vi "initialise.vi"(8 "error in (no error)":errorcluster, 11 "FPGA_AK101022Resonance in":refnum<class "FPGAWrapperAK101022Resonance.lvclass">) -> (0 "error out":errorcluster, 3 "FPGA_AK101022Resonance out":refnum<class "FPGAWrapperAK101022Resonance.lvclass">)   [LabVIEW 2010, in "FPGAWrapperAK101022Resonance.lvclass"]
uses:
  FPGAWrapperAK101022Resonance.lvclass
  GenericFPGAWrapper/GenericFPGAWrapper/GenericFPGAWrapper.lvclass
  scan_specification_cluster.ctl
  grabber/config_data_cluster.ctl
  FPGAWrapperAK101022Resonance.lvclass/FPGAWrapperAK101022Resonance.ctl
  class_data.vi
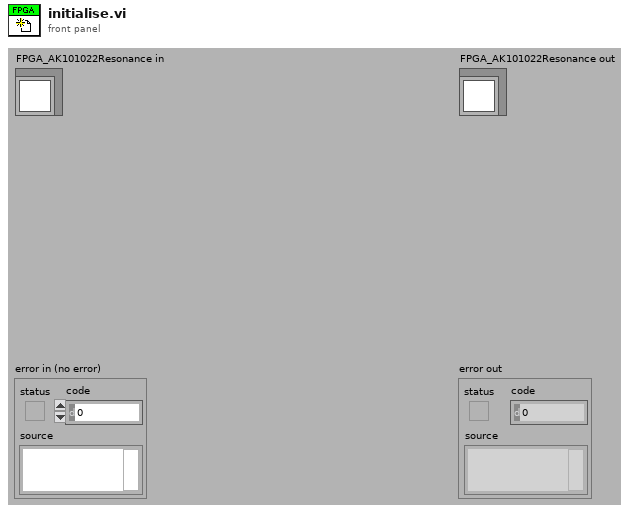
[diagram p1: front panel]
types:
  T1 = typedef "scan_specification_cluster.ctl" = cluster{"x amplitude":u16, "x resolution (pixels)":u16, "x offset fly-forward (iterations)":u16, "x offset fly-back (iterations)":u16, "y resolution (nr. of lines)":u16, "y step size":u16, "iterations per pixel":u16, "number of frames":i32, "y offset (pixels)":u16, "number of y-brake lines  (before y-fly-back)":u16, "number y-brake lines (after y-fly-back)":u16, "number of y-fly-back steps":u16, "lines per z step":u16, "number of z/intensity tuples":u16}
  T2 = typedef "config_data_cluster.ctl" = cluster{"channel offsets":u32[], "invert channel?":bool[], "ADC clock phase":i32}
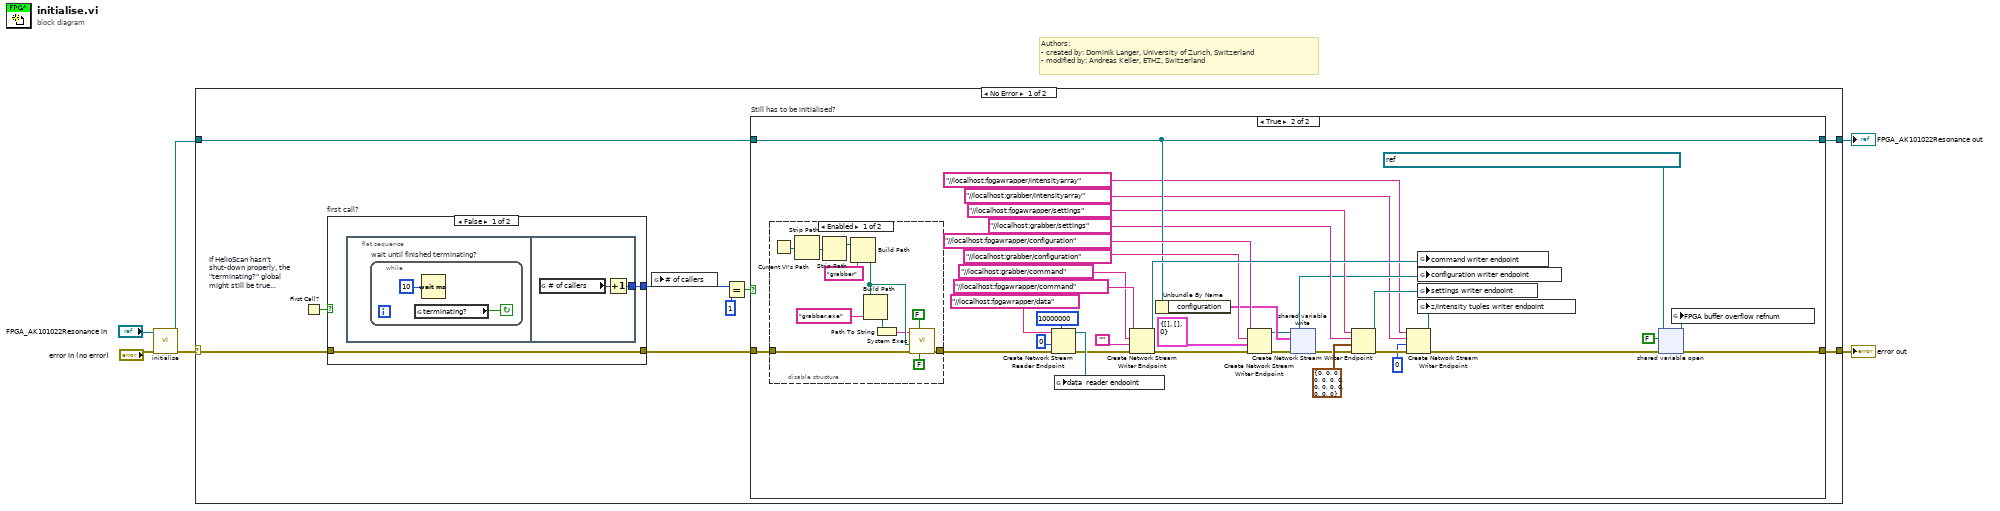
[diagram p0: block diagram]
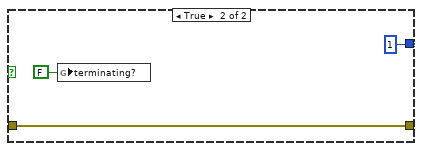
[diagram p2: hidden frame]
diagram:
  # "Authors: \n- created by: Dominik Langer, University of Zurich, Switzerland\n- modified by: Andreas Keller, ETHZ, Switzerland"
  n1 = call-parent "initialise.vi"("error in (no error)"="error in (no error)", "GenericPlugin in"="FPGA_AK101022Resonance in") -> ("error out"=w2:errorcluster, "GenericPlugin out"=w1:refnum<class "FPGAWrapperAK101022Resonance.lvclass">)  [unwired: 8 in]
  n2 = case shown="No Error" w2 {
    selector: w2 -> [w8 w76]
    tunnel: [w15 w76] -> w6
    tunnel: w1 -> [w7 w75]
    tunnel: [w9 w75] -> w5
    frame No Error {
      n3 = First Call? "If HelioScan hasn't shut-down properly, the \"terminating?\" global might still be true..."() -> (First Call?: T/F=w14:bool)
      n4 = case "first call?" shown="False" w14 {
        tunnel: [w17 1 ("# of callers")] -> w12
        tunnel: [w16 w23] -> w13
        tunnel: w8 -> [w16 w23]
        frame False {
          n5 = flat-sequence {
            tunnel: [w21] -> w17
            frame #0 {
              n6 = while "wait until finished terminating?" {
                stop <- w18 continue-if-true
                n7 = global read "class_data.vi" "terminating?"() -> (w18:bool)
                n8 = Wait (ms)(milliseconds to wait=u32 10) -> ()  [unwired: 1 out]
              }
            }
            frame #1 {
              n9 = global read "class_data.vi" "# of callers"() -> (w20:i32)
              n10 = Increment(x=w20) -> (x+1=w21:i32)
            }
          }
        }
        frame True {
          n11 = global write "class_data.vi" "terminating?"(FALSE ("terminating?")) -> ()
        }
      }
      n12 = global write "class_data.vi" "# of callers"(w12) -> ()
      n13 = Equal?(x=w12, y=1) -> (x = y?=w10:bool)
      n14 = case "Still has to be initialised?" shown="True" w10 {
        tunnel: w13 -> [w26 w61]
        tunnel: [w26 w45] -> w15
        tunnel: w7 -> [w25 w42]
        tunnel: [w25 w42] -> w9
        frame False {
        }
        frame True {
          n15 = disable-structure shown="Enabled" {
            disable-tunnel: w61 -> [w66 w74]
            disable-tunnel: [w65 w74] -> w53
            frame Enabled {
              n16 = Current VI's Path() -> (path=w64:path)
              n17 = Strip Path(path=w64) -> (stripped path=w63:path)  [unwired: 1 out]
              n18 = Strip Path(path=w63) -> (stripped path=w62:path)  [unwired: 1 out]
              n19 = Build Path(base path=w62, name or relative path="grabber") -> (appended path=w71:path)
              n20 = Build Path(base path=w71, name or relative path="grabber.exe" ("command line")) -> (appended path=w70:path)
              n21 = Path To String(path=w70) -> (string=w69:string)
              n22 = call <vilib>:"System Exec.vi"("run minimized? (F)"=FALSE, "wait until completion? (T)"=FALSE, "error in (no error)"=w66, "working directory"=w71, "command line"=w69) -> ("error out"=w65:errorcluster)  [unwired: 3 in, 3 out]
            }
            frame Disabled {
            }
          }
          n23 = Create Network Stream Reader Endpoint(7:10000000 ("reader buffer size"), 8:w53, 9:u32 0, 11:"//localhost:fpgawrapper/data" ("writer name")) -> (0:w50:errorcluster, 3:w58:refnum<k21>)  [unwired: 2 in]
          n24 = global write "class_data.vi" "data  reader endpoint"(w58) -> ()
          n25 = Create Network Stream Writer Endpoint(8:w50, 9:"", 10:"//localhost:grabber/command" ("reader url"), 11:"//localhost:fpgawrapper/command" ("writer name")) -> (0:w47:errorcluster, 3:w49:refnum<k21>)  [unwired: 2 in]
          n26 = Unbundle By Name(w42) -> ("configuration"=w41:T2)
          n27 = Create Network Stream Writer Endpoint(8:w47, 9:T2 {"channel offsets"=[], "invert channel?"=[], "ADC clock phase"=0} ("configuration"), 10:"//localhost:grabber/configuration" ("reader url"), 11:"//localhost:fpgawrapper/configuration" ("writer name")) -> (0:w36:errorcluster, 3:w34:refnum<k21>)  [unwired: 2 in]
          n28 = shared-variable-write(w34, w36, w41) -> (w38:refnum<k21>, w35:errorcluster)  [unwired: 1 in, 1 out]
          n29 = Create Network Stream Writer Endpoint(8:w35, 9:T1 {"x amplitude"=0, "x resolution (pixels)"=0, "x offset fly-forward (iterations)"=0, "x offset fly-back (iterations)"=0, "y resolution (nr. of lines)"=0, "y step size"=0, "iterations per pixel"=0, "number of frames"=0, "y offset (pixels)"=0, "number of y-brake lines  (before y-fly-back)"=0, "number y-brake lines (after y-fly-back)"=0, "number of y-fly-back steps"=0, "lines per z step"=0, "number of z/intensity tuples"=0} ("scan specification"), 10:"//localhost:grabber/settings" ("reader url"), 11:"//localhost:fpgawrapper/settings" ("writer name")) -> (0:w32:errorcluster, 3:w33:refnum<k21>)  [unwired: 2 in]
          n30 = Create Network Stream Writer Endpoint(8:w32, 9:u32 0, 10:"//localhost:grabber/intensityarray" ("reader url"), 11:"//localhost:fpgawrapper/intensityarray" ("writer name")) -> (0:w31:errorcluster, 3:w27:refnum<k21>)  [unwired: 2 in]
          n31 = global write "class_data.vi" "command writer endpoint"(w49) -> ()
          n32 = global write "class_data.vi" "configuration writer endpoint"(w38) -> ()
          n33 = global write "class_data.vi" "settings writer endpoint"(w33) -> ()
          n34 = global write "class_data.vi" "z/intensity tuples writer endpoint"(w27) -> ()
          n35 = shared-variable-open(refnum<k21> "ni.var.psp://localhost/grabber variables/FPGA buffer overflow%3F" ("shared variable refnum in"), w31, FALSE) -> (w54:refnum<k21>, w45:errorcluster)  [unwired: 1 in]
          n36 = global write "class_data.vi" "FPGA buffer overflow refnum"(w54) -> ()
        }
      }
    }
    frame Error {
    }
  }
  "error out" <- w6
  "FPGA_AK101022Resonance out" <- w5
